vi "GetThisLevelConfiguration.vi"(8 "error in (no error)":errorcluster, 11 "SMO":refnum<class "SMO.lvclass">) -> (0 "error out":errorcluster, 2 "Configuration":variant, 3 "SMO out":refnum<class "SMO.lvclass">)   [LabVIEW 2013, in "SMO.lvclass"]
uses:
  SMO.lvclass
  Support/Attribute.Config/Attribute.Config.lvclass
  Support/Attribute/Attribute.lvclass
panel:
  # "For instructions on how to use the JKI State Machine Objects, examples and video tutorials, visit:\nhttp://jki.net/state-machine-objects/\n\nJKI State Machine Objects™\nhttp://jki.net/state-machine-objects/\nCopyright (C) 2005-2015, JKI <info@jki.net>\nALL RIGHTS RESERVED"
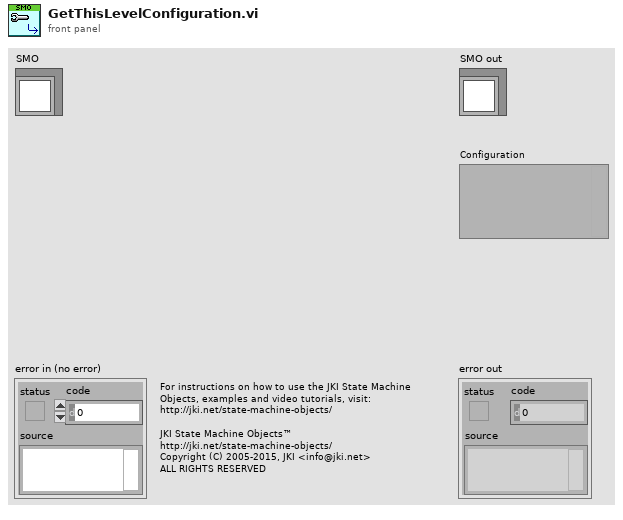
[diagram p1: front panel]
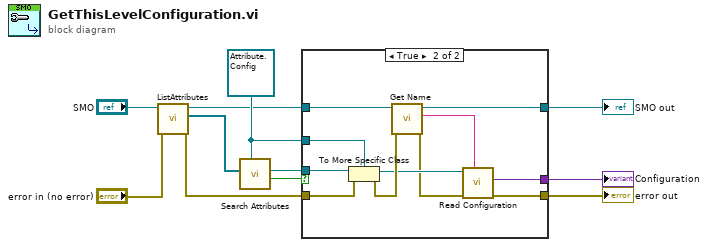
[diagram p0: block diagram]
diagram:
  w10 = refnum<class "Attribute.Config.lvclass"> refnum ("Attribute.Config.lvclass")
  n1 = call "ListAttributes.vi"("error in (no error)"="error in (no error)", "SMO in"="SMO") -> ("error out"=w7:errorcluster, "[Attributes]"=w5:refnum<class "Attribute.lvclass">[], "SMO out"=w9:refnum<class "SMO.lvclass">)  [unwired: 7 in]
  n2 = call "Search Attributes.vi"("Attribute type"=w10, "[Attributes]"=w5) -> ("found"=w3:bool, "Attribute out"=w11:refnum<class "Attribute.lvclass">)  [unwired: 8 in]
  n3 = case shown="True" w3 {
    tunnel: w11 -> [_ w24]
    tunnel: w10 -> [_ w23]
    tunnel: w9 -> [w13 w22]
    tunnel: [w13 w21] -> w8
    tunnel: w7 -> [w12 w19]
    tunnel: [w12 w17] -> w2
    tunnel: [_ w16] -> w1
    frame False {
    }
    frame True {
      n4 = To More Specific Class(target class=w23, reference=w24, error in=w19) -> (specific class reference=w15:refnum<class "Attribute.Config.lvclass">, error out=w20:errorcluster)
      n5 = call "Get Name.vi"("error in (no error)"=w20, "SMO"=w22) -> ("error out"=w14:errorcluster, "Name"=w18:string, "SMO out"=w21:refnum<class "SMO.lvclass">)  [unwired: 7 in]
      n6 = call-dynamic "Read Configuration.vi"("Name"=w18, "error in (no error)"=w14, "Attribute.Config in"=w15) -> ("error out"=w17:errorcluster, "Configuration"=w16:variant)  [unwired: 6 in, 1 out]
    }
  }
  "error out" <- w2
  "SMO out" <- w8
  "Configuration" <- w1
